vi "CD Init.vi"(8 "Error (in)":errorcluster, 11 "Device Reference":T16 format="%.0x") -> (0 "Error (out)":errorcluster, 1 "Inline Status Channels Refs":T3[](array[typedef]) format="%.0x", 2 "Card Parameters (out)":T18, 3 "Output Channel Data []":T7[](array[typedef]) {"Labels Settings"."Label Timestamp Channel Data Reference" format="%.0x"; "Labels Settings"."Label Disable/Trigger Channel Reference" format="%.0x"; "Labels Settings"."Word"."Param Setting"."Item Refs" format="%.0x"; "Labels Settings"."Word"."Param Setting"."Num Bits" min=1 max=32; "Labels Settings"."Word"."Param Setting"."Start Bit" min=8 max=31; "Labels Settings"."Label" format="%.0o"}, 4 "Input Channel Data []":T7[](array[typedef]) {"Labels Settings"."Label Timestamp Channel Data Reference" format="%.0x"; "Labels Settings"."Label Disable/Trigger Channel Reference" format="%.0x"; "Labels Settings"."Word"."Param Setting"."Item Refs" format="%.0x"; "Labels Settings"."Word"."Param Setting"."Num Bits" min=1 max=32; "Labels Settings"."Word"."Param Setting"."Start Bit" min=8 max=31; "Labels Settings"."Label" format="%.0o"}, 6 "Maps":T1 {"Tx Map - Acyclic Labels - Parameters Channels"."Channel Data Reference" format="%.0x"; "Tx Map - Trigger Channels"."Channel Data Reference" format="%.0x"; "Tx Map - Cyclic Labels - Parameters Channels"."Channel Data Reference" format="%.0x"; "Tx Map - Disable Channels"."Channel Data Reference" format="%.0x"})   [LabVIEW 2020, in "Ballard Arinc-429 Engine.lvlib"]
doc: "This VI reads all properties, creates different Maps (Tx) and initializes the Core of the board using XML file. Initialization is done here because Rx part is done Inline and Tx part asynchronously."
uses:
  Ballard Arinc-429 Engine.lvlib
  <vilib>/NI VeriStand/Custom Device API/Custom Device Item Ref.ctl
  RT Controls/Card Parameters.ctl
  Shared/Controls and Global/Initialization Method.ctl
  Shared/Controls and Global/RT HW Channel.ctl
  Shared/Controls and Global/RT Label Settings.ctl
  Shared/Controls and Global/Label.ctl
  Shared/Controls and Global/transferPeriod.ctl
  Shared/Controls and Global/RT Word Settings.ctl
  Shared/Controls and Global/RT Param Setting.ctl
  Shared/Controls and Global/Start Bit.ctl
  Shared/Controls and Global/Number of Bits.ctl
  <vilib>/NI VeriStand/Custom Device API/Block Data Reference.ctl
  <vilib>/NI VeriStand/Custom Device API/Data Reference.ctl
  Shared/Controls and Global/TransferType.ctl
  RT Controls/Tx_Maps.ctl
  RT Controls/RT Tx Association.ctl
  RT Controls/RT Tx Default Raw Value.ctl
  RT Controls/RT Tx Default Raw Value_Association.ctl
  RT Controls/RT Tx Association Trigger Channels.ctl
  RT Controls/RT Init States.ctl
  <vilib>/NI VeriStand/Custom Device API/Custom Device Channel Type.ctl
  Shared/Controls and Global/Compiled.Settings.ctl
  Shared/Controls and Global/Global.vi
  <vilib>/NI VeriStand/Custom Device API/Get Item Property (I32).vi
  <vilib>/NI VeriStand/Custom Device API/Get Item Property (U16).vi
  <vilib>/NI VeriStand/Custom Device API/Get Item Property (Variant).vi
  <vilib>/NI VeriStand/Custom Device API/Custom Device API.lvlib
  Shared/Ballard Arinc-429 Shared.lvlib
  <vilib>/NI VeriStand/Custom Device Tools/Custom Device Utility Library/Custom Device Utility Library.lvlib
panel:
  out "# of Input Channels":i32
  out "# of Output Channels":i32
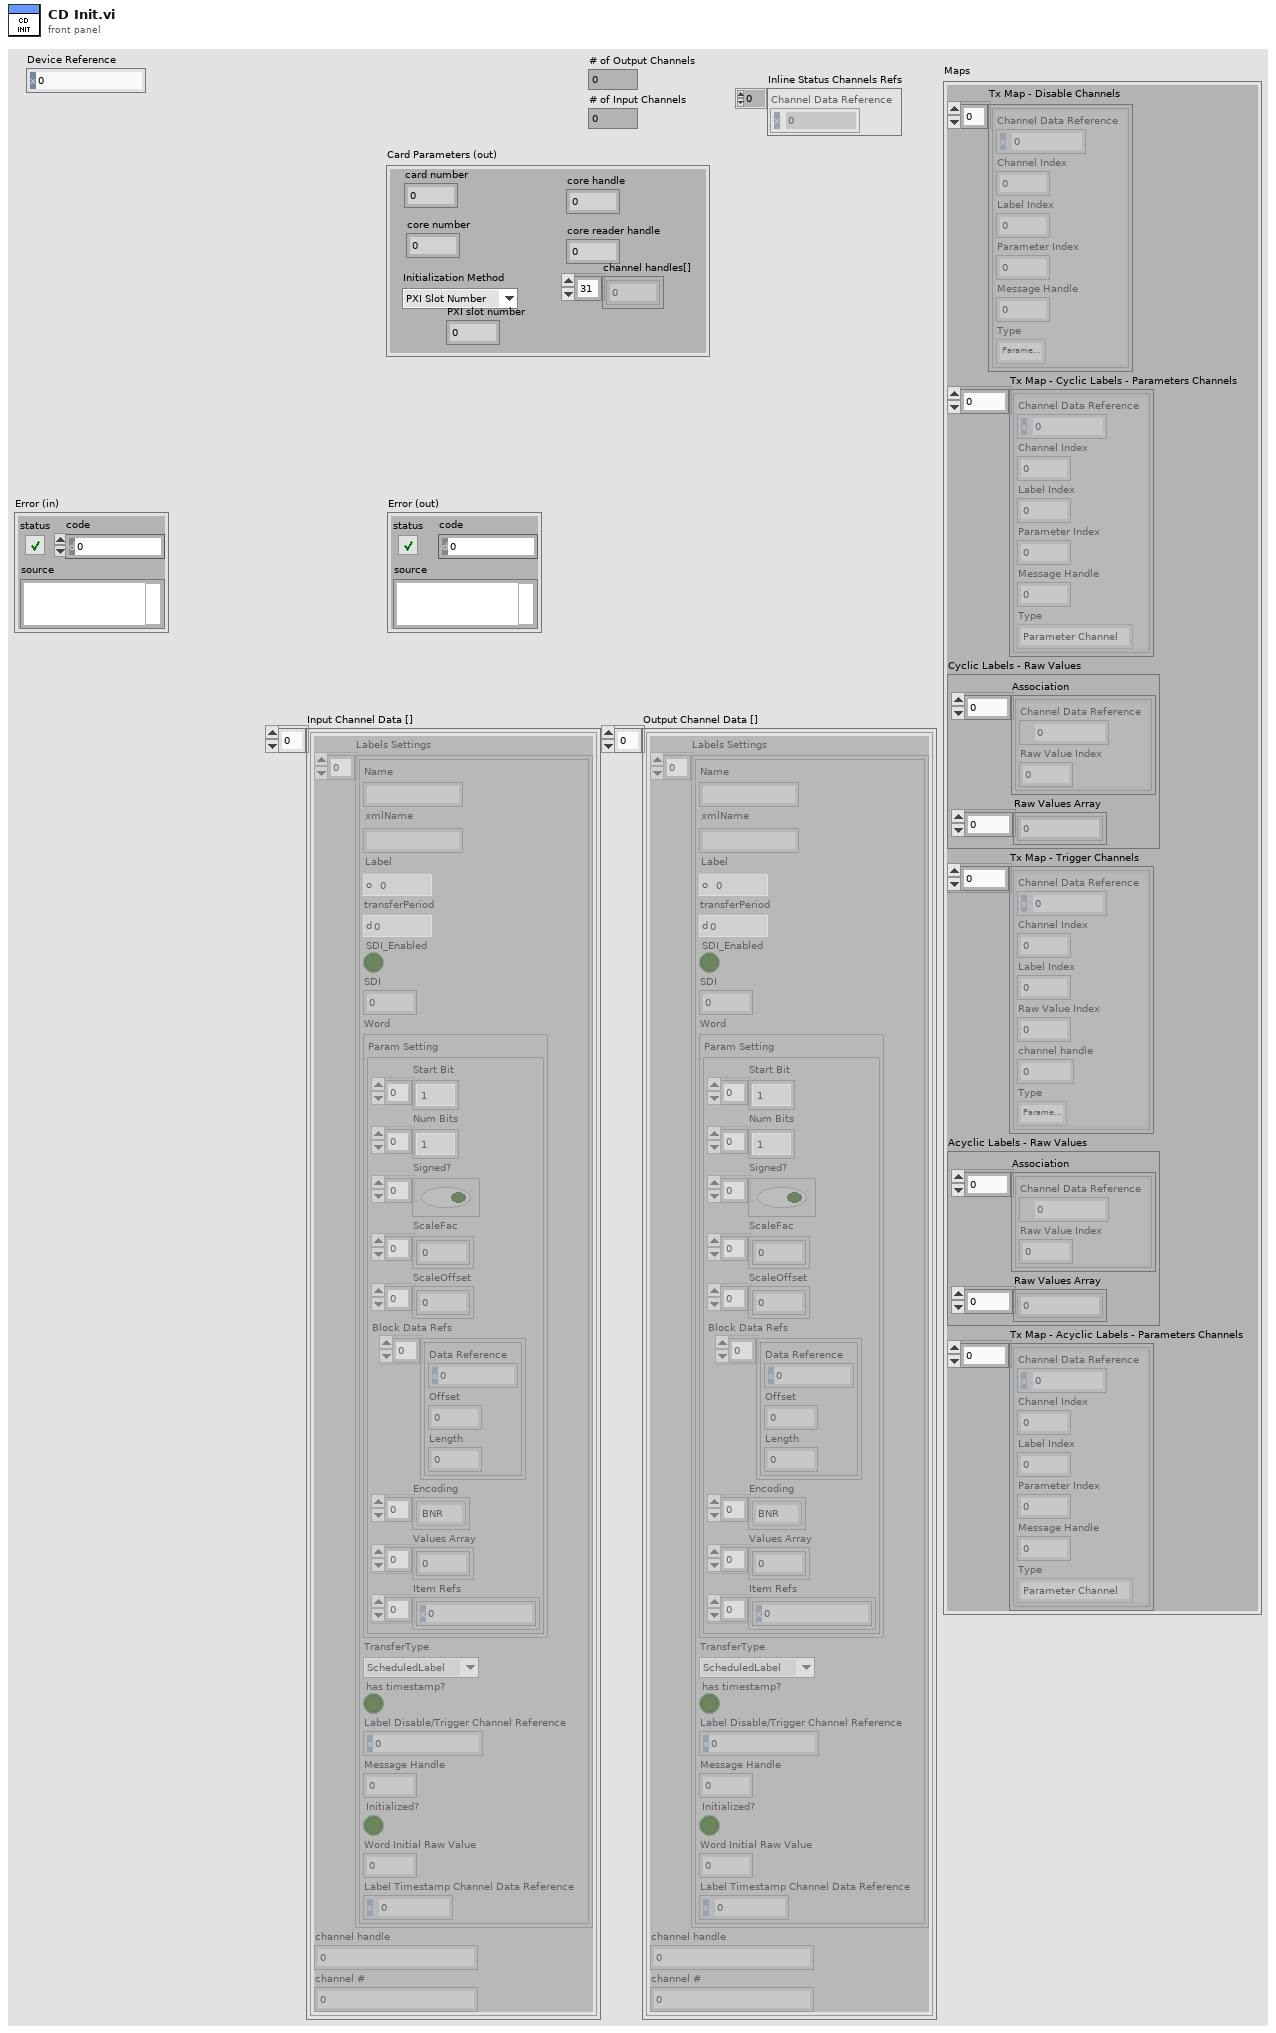
[diagram p1: front panel]
types:
  T1 = typedef "Ballard Arinc-429 Engine.lvlib/Tx_Maps.ctl" = cluster{"Tx Map - Disable Channels":T2[], "Tx Map - Cyclic Labels - Parameters Channels":T2[], "Cyclic Labels - Raw Values":T4, "Tx Map - Trigger Channels":T6[], "Acyclic Labels - Raw Values":T4, "Tx Map - Acyclic Labels - Parameters Channels":T2[]}
  T2 = typedef "Ballard Arinc-429 Engine.lvlib/RT Tx Association.ctl" = cluster{"Channel Data Reference":T3, "Channel Index":i32, "Label Index":i32, "Parameter Index":i32, "Message Handle":u64, "Type":enum16{"Parameter Channel", "Disable/Trigger Channel"}}
  T3 = typedef "Custom Device API.lvlib/Data Reference.ctl" = i32
  T4 = typedef "Ballard Arinc-429 Engine.lvlib/RT Tx Default Raw Value.ctl" = cluster{"Association":T5[], "Raw Values Array":u32[]}
  T5 = typedef "Ballard Arinc-429 Engine.lvlib/RT Tx Default Raw Value_Association.ctl" = cluster{"Channel Data Reference":T3, "Raw Value Index":i32}
  T6 = typedef "Ballard Arinc-429 Engine.lvlib/RT Tx Association Trigger Channels.ctl" = cluster{"Channel Data Reference":T3, "Channel Index":i32, "Label Index":i32, "Raw Value Index":i32, "channel handle":u64, "Type":enum16{"Parameter Channel", "Disable/Trigger Channel"}}
  T7 = typedef "Ballard Arinc-429 Shared.lvlib/RT HW Channel.ctl" = cluster{"Labels Settings":T8[], "channel handle":u64, "channel #":u16}
  T8 = typedef "Ballard Arinc-429 Shared.lvlib/RT Label Settings.ctl" = cluster{"Name":string, "xmlName":string, "Label":T9, "transferPeriod":T10, "SDI_Enabled":bool, "SDI":u8, "Word":T11, "TransferType":T17, "has timestamp?":bool, "Label Disable/Trigger Channel Reference":T16, "Message Handle":u64, "Initialized?":bool, "Word Initial Raw Value":u32, "Label Timestamp Channel Data Reference":T3}
  T9 = typedef "Ballard Arinc-429 Shared.lvlib/Label.ctl" = u8
  T10 = typedef "Ballard Arinc-429 Shared.lvlib/transferPeriod.ctl" = u32
  T11 = typedef "Ballard Arinc-429 Shared.lvlib/RT Word Settings.ctl" = cluster{"Param Setting":T12}
  T12 = typedef "Ballard Arinc-429 Shared.lvlib/RT Param Setting.ctl" = cluster{"Start Bit":T13[], "Num Bits":T14[], "Signed?":bool[], "ScaleFac":dbl[], "ScaleOffset":dbl[], "Block Data Refs":T15[], "Encoding":enum16{"BNR", "BCD", "Discrete"}[], "Values Array":dbl[], "Item Refs":T16[]}
  T13 = typedef "Ballard Arinc-429 Shared.lvlib/Start Bit.ctl" = i32
  T14 = typedef "Ballard Arinc-429 Shared.lvlib/Number of Bits.ctl" = i32
  T15 = typedef "Custom Device API.lvlib/Block Data Reference.ctl" = cluster{"Data Reference":T3, "Offset":u64, "Length":u64}
  T16 = typedef "Custom Device API.lvlib/Custom Device Item Ref.ctl" = u64
  T17 = typedef "Ballard Arinc-429 Shared.lvlib/TransferType.ctl" = enum16{"ScheduledLabel", "Acyclic", "Block", "Strobe"}
  T18 = typedef "Ballard Arinc-429 Engine.lvlib/Card Parameters.ctl" = cluster{"card number":i32, "core number":i32, "core handle":u64, "core reader handle":u64, "channel handles[]":u64[], "Initialization Method":T19, "PXI slot number":i32}
  T19 = typedef "Ballard Arinc-429 Shared.lvlib/Initialization Method.ctl" = enum16{"PXI Slot Number", "Card Number"}
  T20 = typedef "Ballard Arinc-429 Engine.lvlib/RT Init States.ctl" = enum16{"Initialization", "Get Card Settings", "Get Channel Count", "Parse Channels", "Ballard-429 Initialize", "Get Status Channels Reference", "Exit"}
  T21 = typedef "Custom Device API.lvlib/Custom Device Channel Type.ctl" = enum16{"Input", "Output"}
  T22 = typedef "Ballard Arinc-429 Shared.lvlib/Compiled.Settings.ctl" = cluster{"Name":string, "Rx Config":T7[], "Tx Config":T7[]}
  T23 = typedef "Custom Device API.lvlib/Custom Device File Dependency.ctl" = cluster{"Source":T24, "RT Destination":path, "ForceDownload?":bool, "SupportedTarget":T26, "Version":string}
  T24 = typedef "Custom Device API.lvlib/Path Specification.ctl" = cluster{"Path":path, "Type":T25}
  T25 = typedef "Custom Device API.lvlib/Path Type.ctl" = enum16{"Absolute", "To Base", "To Common Data Dir", "To Application Data Dir"}
  T26 = typedef "Custom Device API.lvlib/Custom Device Supported Target.ctl" = enum16{"All", "PharLap", "VxWorks", "Windows", "Linux_32_ARM", "Linux_x64", "PharLap & Windows", "PharLap & VxWorks", "VxWorks & Windows"}
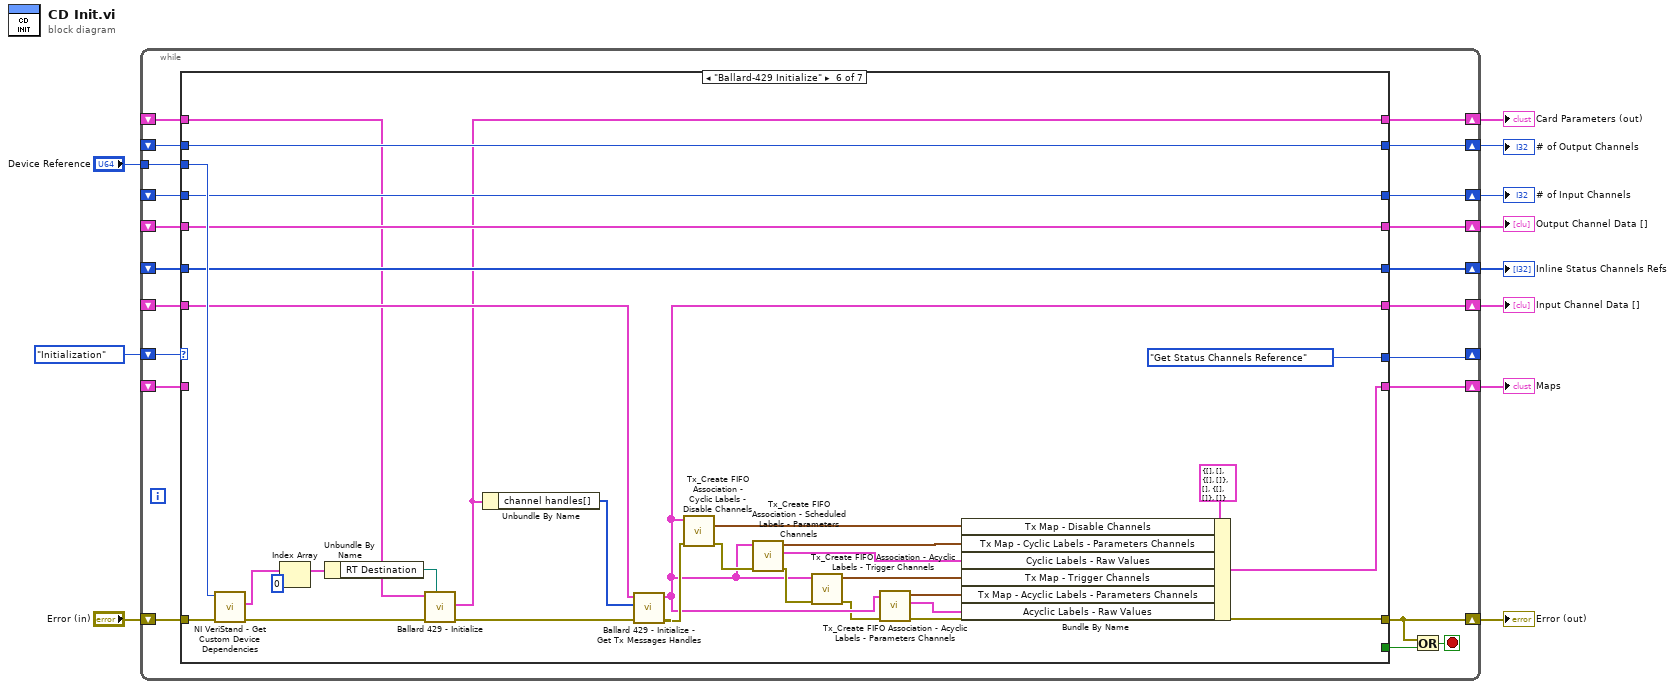
[diagram p0: block diagram]
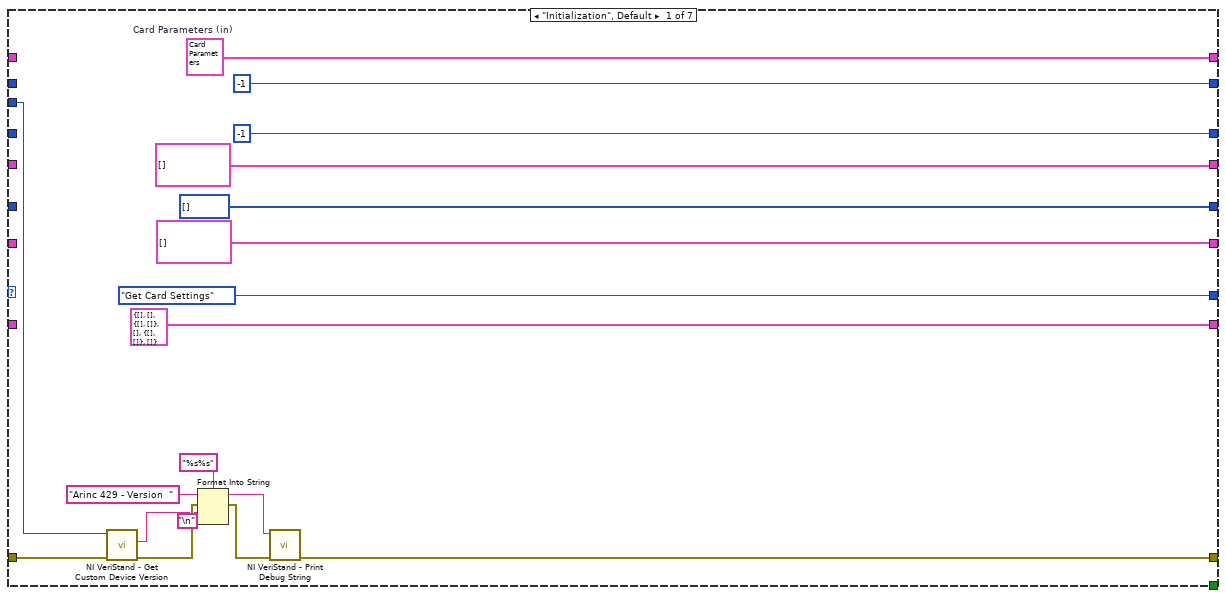
[diagram p2: hidden frame]
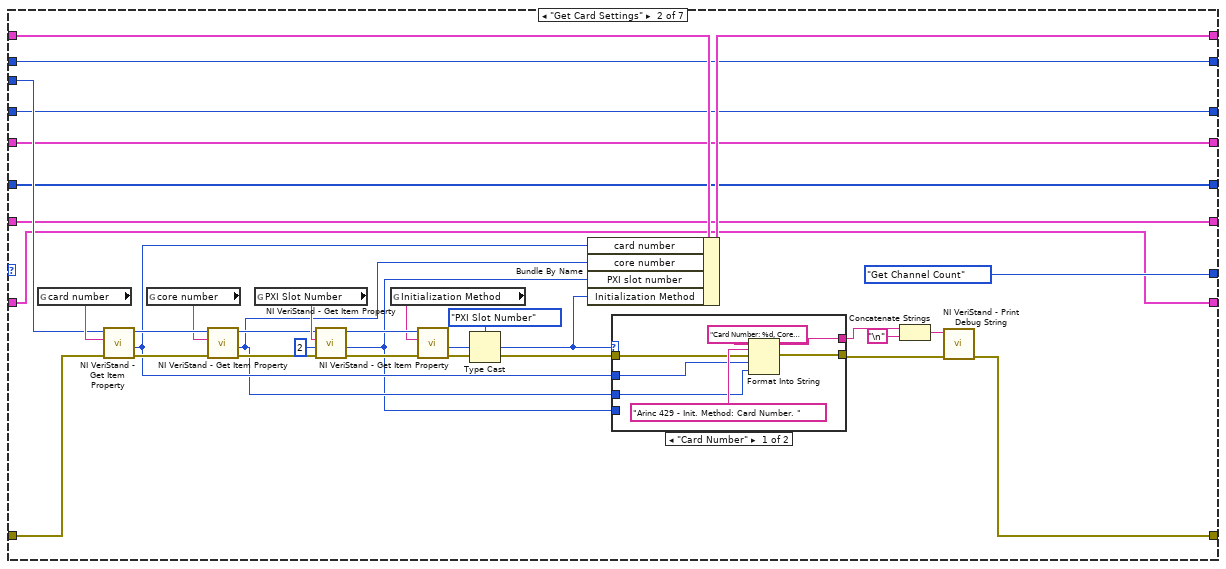
[diagram p3: hidden frame]
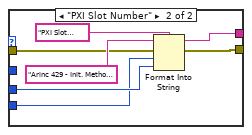
[diagram p4: hidden frame]
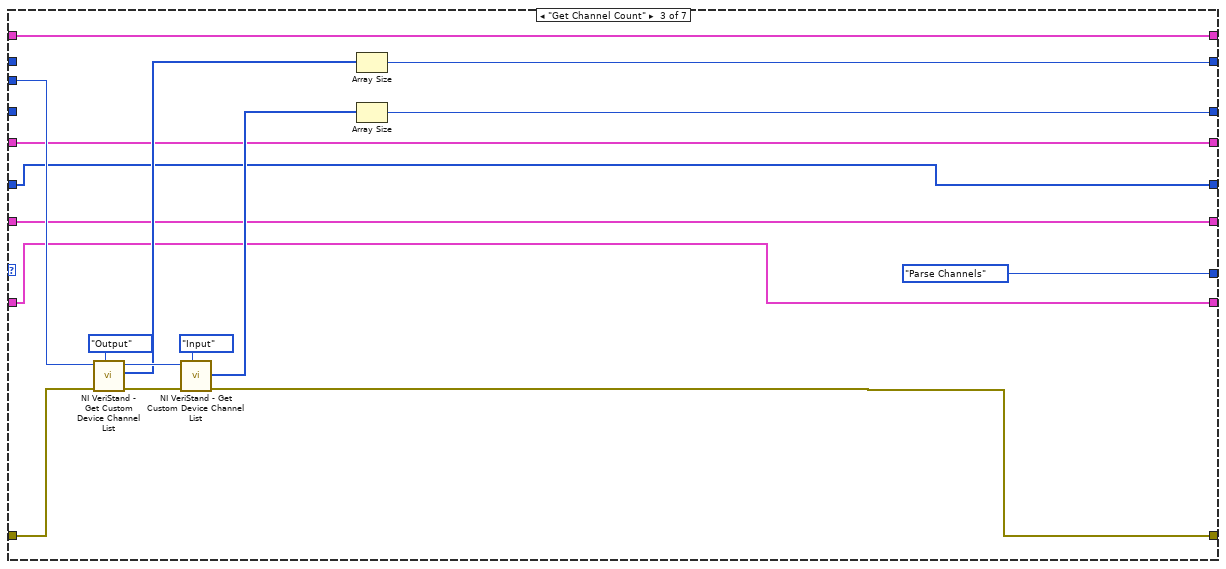
[diagram p5: hidden frame]
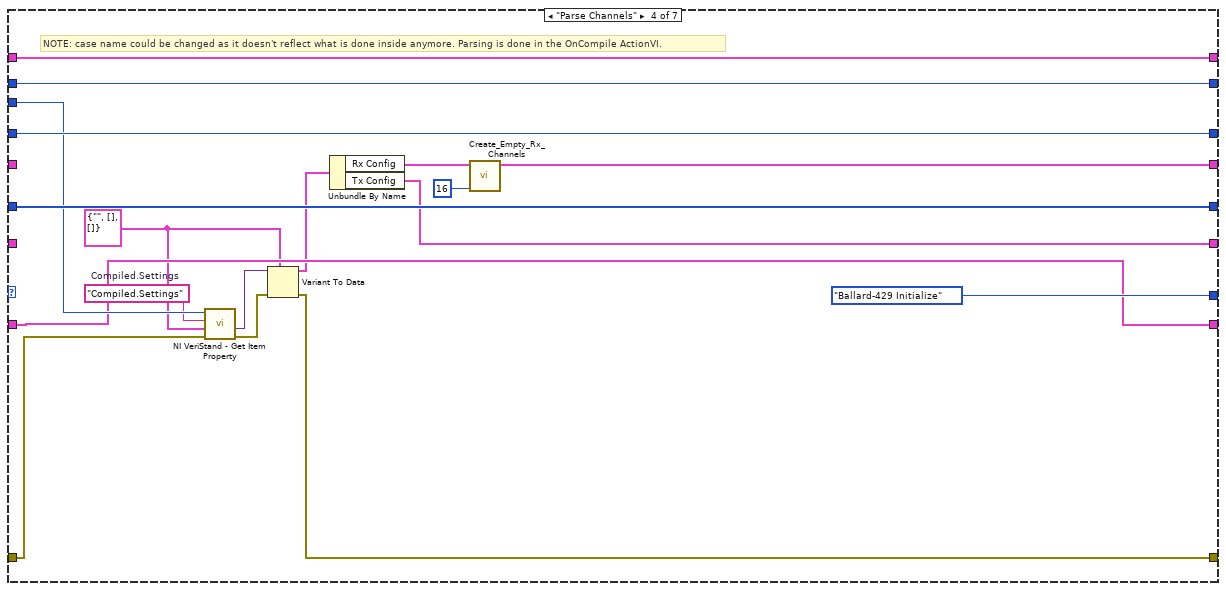
[diagram p6: hidden frame]
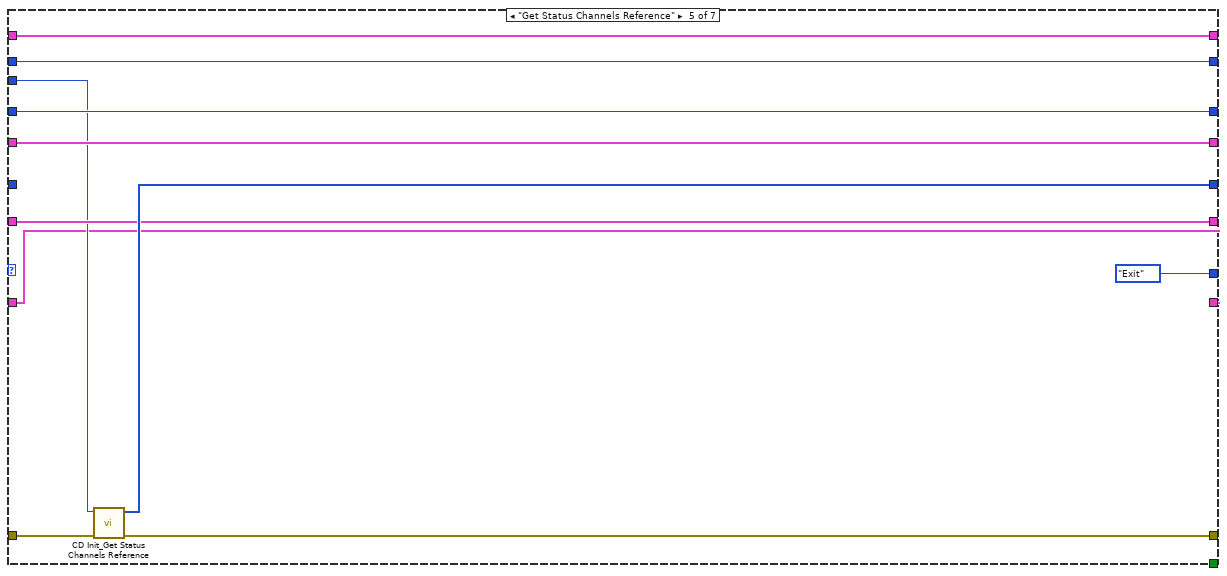
[diagram p7: hidden frame]
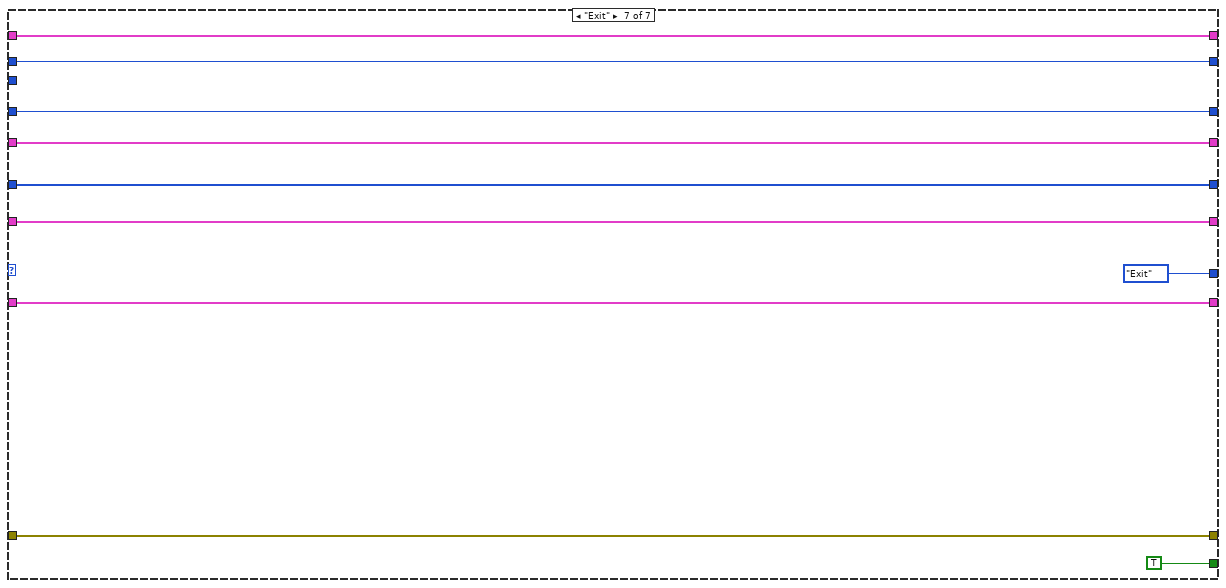
[diagram p8: hidden frame]
diagram:
  n1 = while {
    shift-right: [w31] -> _
    shift-left: RT_Init_States."Initialization" -> [w25]
    tunnel: "Device Reference" -> [w30]
    shift-right: [w26] -> w7
    shift-left: _ -> [w27]
    shift-right: [w24] -> w6
    shift-left: _ -> [w22]
    shift-right: [w23] -> w5
    shift-left: _ -> [w21]
    shift-right: [w20] -> w4
    shift-left: _ -> [w17]
    shift-right: [w19] -> w3
    shift-left: _ -> [w18]
    shift-right: [w16] -> w2
    shift-left: _ -> [w15]
    shift-right: [w14] -> w9
    shift-left: "Error (in)" -> [w32]
    shift-right: [w13] -> w1
    shift-left: _ -> [w12]
    stop <- w29 stop-if-true
    n2 = case shown="\"Ballard-429 Initialize\"" w25 {
      tunnel: w32 -> [w43 w81 w111 w123 w137 w172 w185]
      tunnel: [w41 w79 w99 w122 w134 w149 w185] -> w14
      tunnel: [RT_Init_States."Get Card Settings" RT_Init_States."Get Channel Count" RT_Init_States."Parse Channels" RT_Init_States."Ballard-429 Initialize" RT_Init_States."Exit" RT_Init_States."Get Status Channels Reference" RT_Init_States."Exit"] -> w31
      tunnel: w30 -> [w42 w77 w110 w126 w136 w171 _]
      tunnel: [_ _ _ _ _ _ TRUE] -> w28
      tunnel: w27 -> [_ w76 w106 w132 w138 w145 w182]
      tunnel: [w49 w75 w106 w132 w138 w164 w182] -> w26
      tunnel: [T7[] [] ("Rx Channels Out") w74 w104 w130 w144 w168 w179] -> w24
      tunnel: [T7[] [] ("Channel Data []") w73 w103 w116 w139 w151 w178] -> w23
      tunnel: w22 -> [_ w74 w104 _ w144 w168 w179]
      tunnel: w21 -> [_ w73 w103 _ w139 w169 w178]
      tunnel: [-1 w71 w105 w128 w143 w167 w180] -> w20
      tunnel: [-1 w72 w101 w129 w142 w166 w181] -> w19
      tunnel: w18 -> [_ w72 _ w129 w142 w166 w181]
      tunnel: w17 -> [_ w71 _ w128 w143 w167 w180]
      tunnel: [i32[] [] w70 w102 w127 w140 w165 w177] -> w16
      tunnel: w15 -> [_ w70 w102 w127 _ w165 w177]
      tunnel: [T1 {"Tx Map - Disable Channels"=[], "Tx Map - Cyclic Labels - Parameters Channels"=[], "Cyclic Labels - Raw Values"={"Association"=[], "Raw Values Array"=[]}, "Tx Map - Trigger Channels"=[], "Acyclic Labels - Raw Values"={"Association"=[], "Raw Values Array"=[]}, "Tx Map - Acyclic Labels - Parameters Channels"=[]} ("Maps") w69 w100 w121 w135 w158 w176] -> w13
      tunnel: w12 -> [_ w69 w100 w121 w135 _ w176]
      frame "Initialization", Default {
        w49 = T18 {"card number"=0, "core number"=0, "core handle"=0, "core reader handle"=0, "channel handles[]"=[], "Initialization Method"=enum."PXI Slot Number", "PXI slot number"=0}  # Card Parameters (in)
        n3 = call <vilib>:"NI VeriStand - Get Custom Device Version.vi"("error in (no error)"=w43, "Device Ref in"=w42) -> ("error out"=w40:errorcluster, "Value"=w37:string)  [unwired: 7 in, 1 out]
        n4 = Format Into String(format string="%s%s", initial string="Arinc 429 - Version  ", error in=w40, w37, "\n") -> (resulting string=w35:string, error out=w39:errorcluster)
        n5 = call <vilib>:"NI VeriStand - Print Debug String.vi"("error in (no error)"=w39, "Message"=w35) -> ("error out"=w41:errorcluster)  [unwired: 9 in]
      }
      frame "Get Card Settings" {
        n6 = global read "Global.vi" "card number"() -> (w82:string)
        n7 = call-poly <vilib>:"NI VeriStand - Get Item Property.vi"("error in (no error)"=w81, "Property Name"=w82, "Item Ref in"=w77) -> ("error out"=w80:errorcluster, "Value"=w55:i32, "Item Ref out"=w84:T16)  [unwired: 5 in, 1 out]
        n8 = global read "Global.vi" "core number"() -> (w83:string)
        n9 = call-poly <vilib>:"NI VeriStand - Get Item Property.vi"("error in (no error)"=w80, "Property Name"=w83, "Item Ref in"=w84) -> ("error out"=w66:errorcluster, "Value"=w54:i32, "Item Ref out"=w67:T16)  [unwired: 5 in, 1 out]
        n10 = global read "Global.vi" "PXI Slot Number"() -> (w68:string)
        n11 = call-poly <vilib>:"NI VeriStand - Get Item Property.vi"("error in (no error)"=w66, "Default Value"=2, "Property Name"=w68, "Item Ref in"=w67) -> ("error out"=w64:errorcluster, "Value"=w53:i32, "Item Ref out"=w63:T16)  [unwired: 4 in, 1 out]
        n12 = global read "Global.vi" "Initialization Method"() -> (w62:string)
        n13 = call-poly <vilib>:"NI VeriStand - Get Item Property.vi"("error in (no error)"=w64, "Property Name"=w62, "Item Ref in"=w63) -> ("error out"=w52:errorcluster, "Value"=w61:u16)  [unwired: 5 in, 2 out]
        n14 = Type Cast(type=Initialization_Method."PXI Slot Number" ("Initialization Method"), x=w61) -> (*(type *) &x=w59:T19)
        n15 = Bundle By Name(cluster=w76, "card number"=w55, "core number"=w54, "PXI slot number"=w53, "Initialization Method"=w59) -> (w75:T18)
        n16 = case shown="\"Card Number\"" w59 {
          tunnel: [w91 w98] -> w56
          tunnel: w55 -> [w88 _]
          tunnel: w54 -> [w87 w95]
          tunnel: w53 -> [_ w94]
          tunnel: w52 -> [w86 w93]
          tunnel: [w85 w92] -> w51
          frame "Card Number" {
            n17 = Format Into String(format string="Card Number: %d, Core Number: %d.", initial string="Arinc 429 - Init. Method: Card Number. " ("String to write"), error in=w86, w88, w87) -> (resulting string=w91:string, error out=w85:errorcluster)
          }
          frame "PXI Slot Number" {
            n18 = Format Into String(format string="PXI Slot Number: %d, Core Number: %d.", initial string="Arinc 429 - Init. Method: PXI Slot Number. " ("String to write"), error in=w93, w94, w95) -> (resulting string=w98:string, error out=w92:errorcluster)
          }
        }
        n19 = Concatenate Strings(w56, "\n") -> (w58:string)
        n20 = call <vilib>:"NI VeriStand - Print Debug String.vi"("error in (no error)"=w51, "Message"=w58) -> ("error out"=w79:errorcluster)  [unwired: 9 in]
      }
      frame "Get Channel Count" {
        n21 = call <vilib>:"NI VeriStand - Get Custom Device Channel List.vi"("Channel Type"=Custom_Device_Channel_Type."Output", "error in (no error)"=w111, "Device Ref in"=w110) -> ("error out"=w113:errorcluster, "Specified Channel Ref List"=w109:T16[], "Device Ref out"=w115:T16)  [unwired: 6 out]
        n22 = call <vilib>:"NI VeriStand - Get Custom Device Channel List.vi"("Channel Type"=Custom_Device_Channel_Type."Input", "error in (no error)"=w113, "Device Ref in"=w115) -> ("error out"=w99:errorcluster, "Specified Channel Ref List"=w108:T16[])  [unwired: 7 out]
        n23 = Array Size(array=w109) -> (size(s)=w101:i32)
        n24 = Array Size(array=w108) -> (size(s)=w105:i32)
      }
      frame "Parse Channels" {
        w120 = "Compiled.Settings"  # Compiled.Settings
        w119 = T22 {"Name"="", "Rx Config"=[], "Tx Config"=[]} ("Compiled.Settings")
        # "NOTE: case name could be changed as it doesn't reflect what is done inside anymore. Parsing is done in the OnCompile ActionVI."
        n25 = call-poly <vilib>:"NI VeriStand - Get Item Property.vi"("error in (no error)"=w123, "Default Value"=w119, "Property Name"=w120, "Item Ref in"=w126) -> ("error out"=w125:errorcluster, "Value"=w124:variant)  [unwired: 4 in, 2 out]
        n26 = Variant To Data(error in=w125, type=w119, Variant=w124) -> (data=w118:T22, error out=w122:errorcluster)
        n27 = Unbundle By Name(w118) -> ("Rx Config"=w117:T7[], "Tx Config"=w116:T7[])
        n28 = call "Create_Empty_Rx_Channels.vi"("Nb Channels"=16, "Rx Channels In"=w117) -> ("Rx Channels Out"=w130:T7[])  [unwired: 9 in]
      }
      frame "Get Status Channels Reference" {
        n29 = call "CD Init_Get Status Channels Reference.vi"("error in (no error)"=w137, "Device Reference"=w136) -> ("error out"=w134:errorcluster, "Array"=w140:T3[])  [unwired: 8 in]
      }
      frame "Ballard-429 Initialize" {
        n30 = call <vilib>:"NI VeriStand - Get Custom Device Dependencies.vi"("error in (no error)"=w172, "Device Ref in"=w171) -> ("error out"=w161:errorcluster, "Dependencies"=w174:T23[])  [unwired: 7 in, 1 out]
        n31 = Index Array(array=w174, index=0) -> (element=w173:T23)
        n32 = Unbundle By Name(w173) -> ("RT Destination"=w170:path)
        n33 = call "Ballard 429 - Initialize.vi"("RT Config Filepath"=w170, "Error (in)"=w161, "Card Parameters (in)"=w145) -> ("Error (out)"=w162:errorcluster, "Card Parameters (out)"=w164:T18)  [unwired: 7 in]
        n34 = Unbundle By Name(w164) -> ("channel handles[]"=w160:u64[])
        n35 = call "Ballard 429 - Initialize - Get Tx Messages Handles.vi"("error in (no error)"=w162, "channel handles[]"=w160, "Tx Config in"=w169) -> ("error out"=w152:errorcluster, "Tx Config out"=w151:T7[])  [unwired: 7 in]
        n36 = call "Tx_Create FIFO Association - Cyclic Labels - Disable Channels.vi"("error in (no error)"=w152, "Input Channel Data []"=w151) -> ("error out"=w154:errorcluster, "Cyclic Labels - Disable Channels Map"=w157:T2[])  [unwired: 8 in]
        n37 = call "Tx_Create FIFO Association - Scheduled Labels - Parameters Channels.vi"("error in (no error)"=w154, "Input Channel Data []"=w151) -> ("error out"=w153:errorcluster, "Raw Values"=w155:T4, "Map"=w156:T2[])  [unwired: 7 in]
        n38 = call "Tx_Create FIFO Association - Acyclic Labels - Trigger Channels.vi"("error in (no error)"=w153, "Input Channel Data []"=w151) -> ("error out"=w150:errorcluster, "Map"=w148:T6[])  [unwired: 8 in]
        n39 = call "Tx_Create FIFO Association - Acyclic Labels - Parameters Channels.vi"("error in (no error)"=w150, "Input Channel Data []"=w151) -> ("error out"=w149:errorcluster, "Raw Values"=w146:T4, "Map"=w147:T2[])  [unwired: 7 in]
        n40 = Bundle By Name(cluster=T1 {"Tx Map - Disable Channels"=[], "Tx Map - Cyclic Labels - Parameters Channels"=[], "Cyclic Labels - Raw Values"={"Association"=[], "Raw Values Array"=[]}, "Tx Map - Trigger Channels"=[], "Acyclic Labels - Raw Values"={"Association"=[], "Raw Values Array"=[]}, "Tx Map - Acyclic Labels - Parameters Channels"=[]} ("Maps"), "Tx Map - Disable Channels"=w157, "Tx Map - Cyclic Labels - Parameters Channels"=w156, "Cyclic Labels - Raw Values"=w155, "Tx Map - Trigger Channels"=w148, "Tx Map - Acyclic Labels - Parameters Channels"=w147, "Acyclic Labels - Raw Values"=w146) -> (w158:T1)
      }
      frame "Exit" {
      }
    }
    n41 = Or(x=w14, y=w28) -> (x .or. y?=w29:bool)
  }
  "Error (out)" <- w9
  "Card Parameters (out)" <- w7
  "Output Channel Data []" <- w6
  "Input Channel Data []" <- w5
  "# of Output Channels" <- w3
  "# of Input Channels" <- w4
  "Inline Status Channels Refs" <- w2
  "Maps" <- w1
